vi "play_FXP_AFMss_LinearDistEst_singleAxis.vi"() -> ()   [LabVIEW 2017]
uses:
  fpga_VIs/fixed-point/typeDefs/FXPControlParams_distEst.ctl
  fpga_fp_interface_lib/fpga_interface_types/boolean_indicators.ctl
  <vilib>/Analysis/Matrix/Datatypes/RealMatrix.ctl
  <vilib>/userdefined/High Color/nirio_resource_hc.ctl
  <vilib>/Utility/error.llb/DialogType.ctl
  <vilib>/Analysis/Matrix/Numeric/Conversions/Matrix To Array - RM.vi
  <vilib>/Utility/file.llb/Read Delimited Spreadsheet (DBL).vi
  <vilib>/FPGAPlugInAG/cRIO-9082/niLvFpga_Open_cRIO-9082.vi
  <vilib>/rvi/interface/common/dynamic/niFpgaDynamicAddResources.vi
  <vilib>/FPGAPlugInAG/Dynamic/niLvFpga_Reset_Dynamic.vi
  <vilib>/rvi/interface/common/niFpgaWaitOnOcc.vi
  <vilib>/Utility/error.llb/Error Cluster From Error Code.vi
  <vilib>/rvi/errors/niLvFpgaAdjustHostInterfaceError.vi
  <vilib>/FPGAPlugInAG/Dynamic/niLvFpga_Run_Dynamic.vi
  <vilib>/RVI Host/nirviSupport.llb/nirviErrorClusterFromErrorCode.vi
  fpga_fp_interface_lib/write_FP_data_to_fpga.vi
  fpga_fp_interface_lib/acquire_FXP_18-5_FIFO_1.vi
  <vilib>/Utility/file.llb/Write To Spreadsheet File (DBL).vi
  <vilib>/Analysis/Matrix/Numeric/Conversions/Array To Matrix - RA2.vi
  <vilib>/FPGAPlugInAG/Dynamic/niLvFpga_Close_Dynamic.vi
  <vilib>/rvi/interface/nirviOpenFPGA/nirviOpenFPGA.xnode
  FPGA Bitfiles/XYpeizocontrol_FPGA_FXPAFMssLinearDistEst_singleAxis.lvbitx
  <vilib>/rvi/interface/nirviMethod/nirviMethod.xnode
  <vilib>/rvi/interface/nirviReadWriteControl/nirviReadWriteControl.xnode
  <vilib>/rvi/interface/nirviCloseFPGA/nirviCloseFPGA.xnode
  <vilib>/rvi/errors/niLvFpgaMergeErrorWithErrorCode.vi
  <vilib>/rvi/interface/Simulation/niFpgaSimulationCallBeginRW.vi
  <vilib>/rvi/interface/nirviMethod/StockFPGA_InlinedMethodWaitForSingleIRQ.vi
  <vilib>/FPGAPlugInAG/Dynamic/niLvFpga_WaitOnIrq_Dynamic.vi
  <vilib>/FPGAPlugInAG/Dynamic/niLvFpga_AcknowledgeIrq_Dynamic.vi
  <vilib>/FPGAPlugInAG/Dynamic/niLvFpga_ConfigureFifo_Dynamic.vi
  <vilib>/Analysis/Matrix/NI_Matrix.lvlib
  <vilib>/FPGAPlugInAG/Dynamic/niLvFpga_WriteFifo_Dynamic.vi
  labview/utils_lib/utils.lvlib
  NiFpgaLv.dll
panel:
  out "elements left":i32=1
  in  "N_hyst":i32
  in  "w_s":T1
  in  "r_s":T1
  in  "TF Order":i32
  in  "den":T1
  in  "num":T1
  in  "Tab Control":T2(tab)
  in  "traj_path":path=path "Z:/mpc-journal/step-exps/traj_data.csv"
  in  "TsTicks":i32=1600
  in  "umax":dbl=1.0 format="%#_13g"
  in  "ymax":dbl=4.0 format="%#_13g"
  in  "Iters":i32=25
  in  "SettleTicks":i32=10
  in  "dry_run":bool=TRUE
  in  "control_data_path":path=path "Z:/mpc-journal/step-exps/FXP_lin_Controls01.csv"
  in  "outputDataPath":path=path "Z:/mpc-journal/step-exps/expOut_multiAxis_tmp.csv"
  out "ControlParams":T3={"umax"=3.0, "Ns_obs/cntrl"=0, "ref_f_VEC"=[0.0, 0.0], "du_max"=0.0}
  in  "ABORT":bool
  out "XY Graph":cluster{dbl[], "2D Data Out":dbl[]}[](graph)
  in  "read_file":bool=TRUE
  in  "All_matrix":T1
  in  "Ns_obs/cntrl":u8=21
  in  "yref":T1
  in  "du_max":dbl=1.0 format="%#_13g"
  out "AllMatrix":dbl[](array[numeric])
  out "ControlMatrices":T4
  out "result_data":T1
  out "boolean  indicators":T5
  out "error out":errorcluster
  out "Empty Elements Remaining":u32
  out "size(s)":i32[](array[numeric])
  out "u_k out":fxp<+/-,32,5>
  # "NOTE: Ns is the number of states in the plant. The number of states in the \nobserver is Ns+1. Thus, for B, L, C, and A, we use NS+1. For K and Xss, we use Ns\nbecause the controller does not operate on the disturbance state, Xd."
  # "yk\nulin\ndu\nu_inv\nIpow\nX"
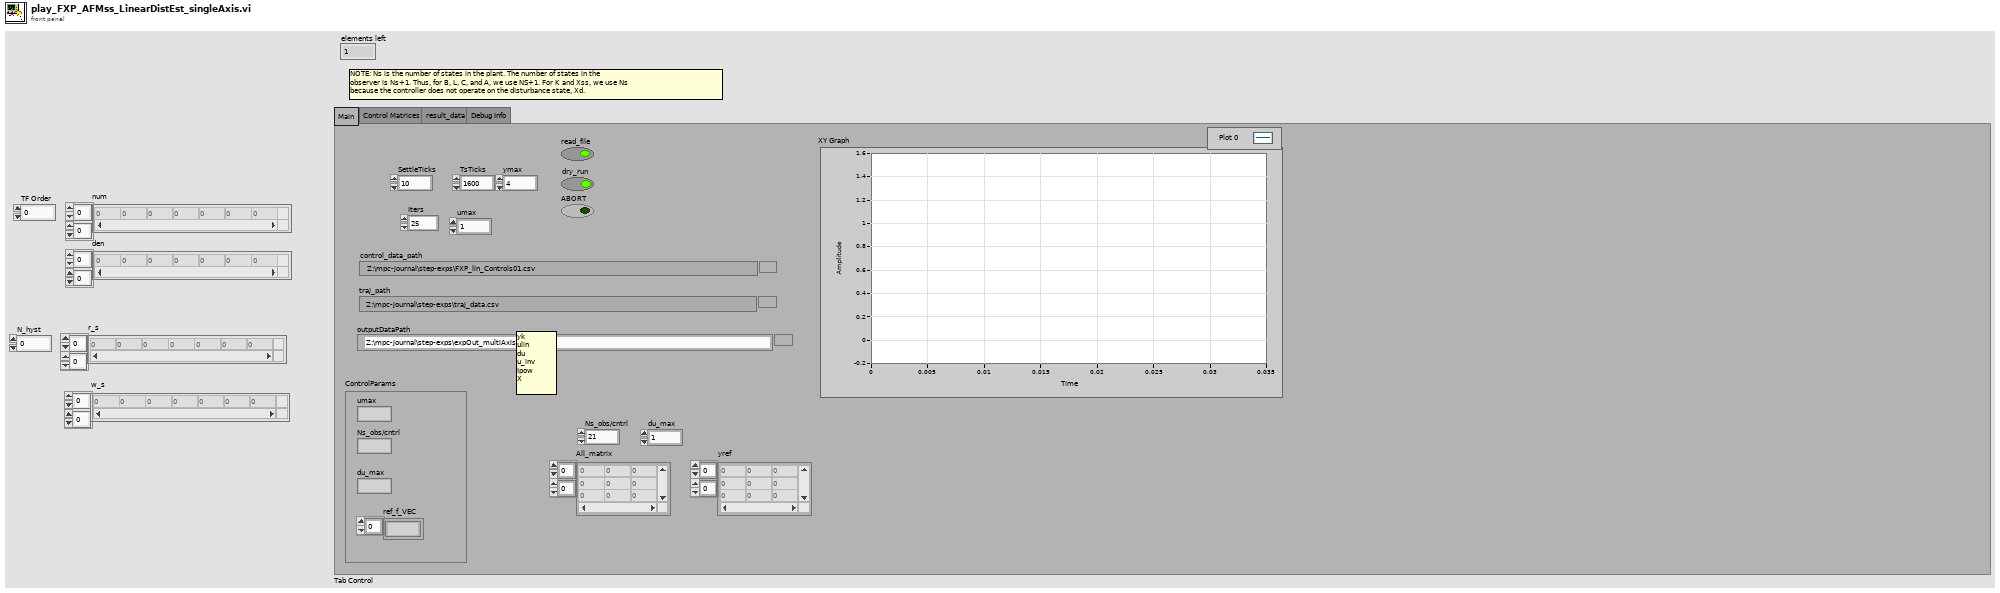
[diagram p1: front panel]
types:
  T1 = typedef "NI_Matrix.lvlib/RealMatrix.ctl" = dbl[][]
  T2 = enum32{"Main", "Control Matrices", "result_data", "Debug Info"}
  T3 = typedef "FXPControlParams_distEst.ctl" = cluster{"umax":fxp<+/-,18,5>, "Ns_obs/cntrl":u8, "ref_f_VEC":fxp<+/-,32,5>[], "du_max":fxp<+/-,18,5>}
  T4 = cluster{"Az":fxp<+/-,32,4>[][], "Bz":dbl[][], "Lz":dbl[][], "Kz":dbl[][], "NxNu":dbl[][]}
  T5 = typedef "boolean_indicators.ctl" = cluster{"unstable-z-traj":bool, "input fifo time-out":bool, "logging fifo timeout":bool, "scanning finished":bool, "unstable-x-traj":bool, "unstable-y-traj":bool, "ABORT":bool, "All Measurements Done":bool, "fpga_finished":bool}
  T6 = typedef "nirio_resource_hc.ctl" = tag
  T7 = typedef "ObserverMatrices.ctl" = cluster{"Az":fxp<+/-,32,4>[][], "Bz":dbl[][], "Lz":dbl[][], "Kz":dbl[][], "NxNu":dbl[][]}
  T8 = cluster{"unstable-z-traj":bool, "input fifo time-out":bool, "logging fifo timeout":bool, "scanning finished":bool, "unstable-x-traj":bool, "unstable-y-traj":bool, "ABORT":bool, "All Measurements Done":bool, "fpga_finished":bool}
  T9 = typedef "DialogType.ctl" = u16
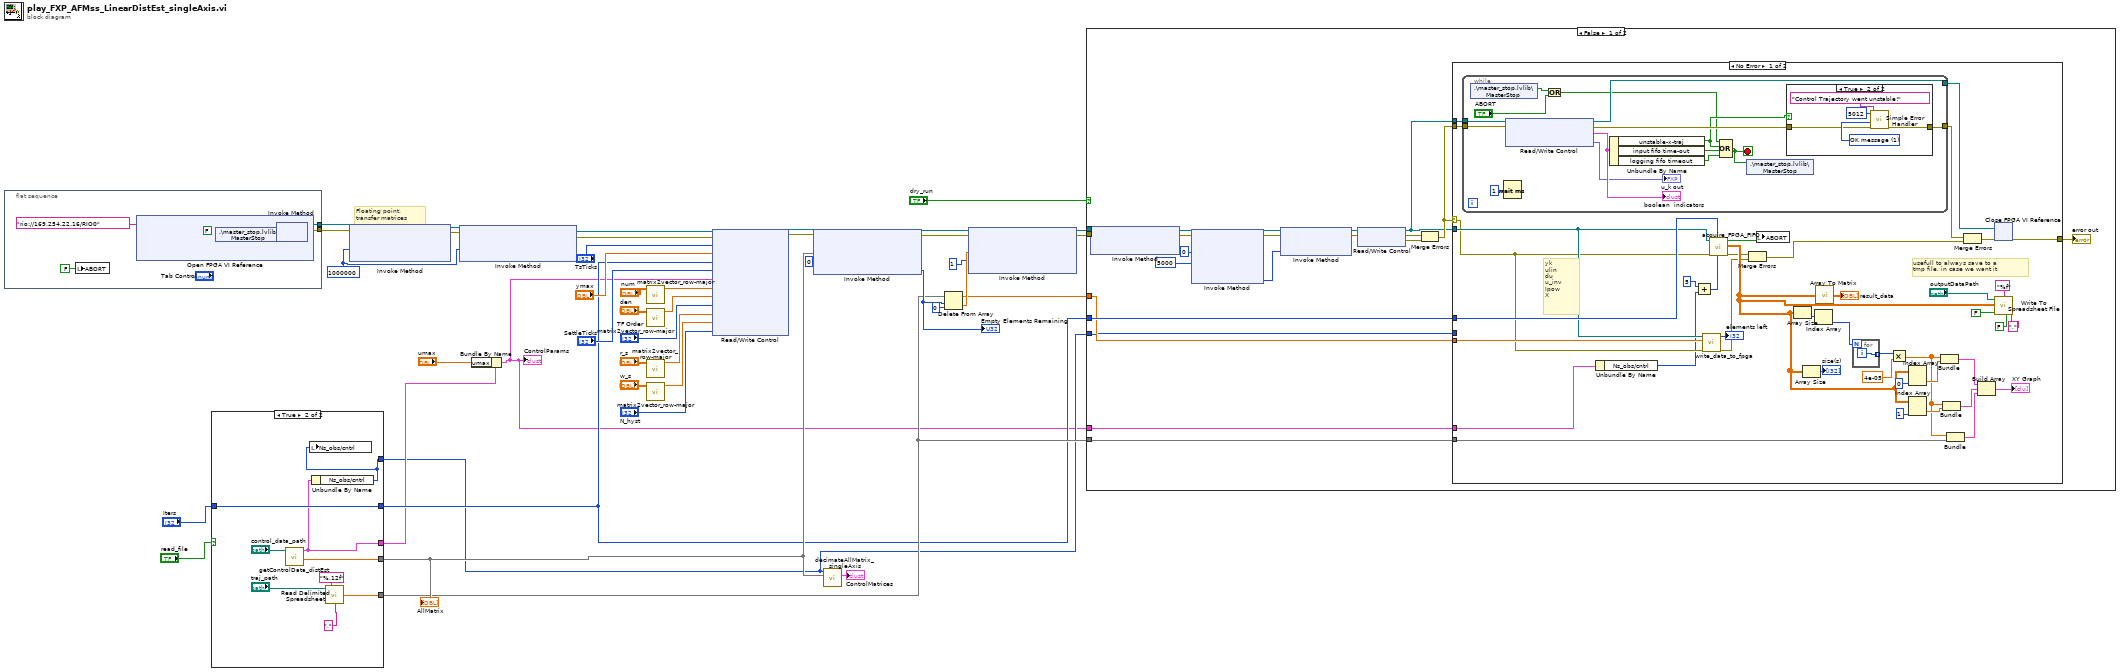
[diagram p0: block diagram]
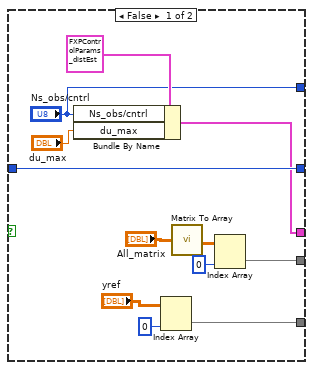
[diagram p2: hidden frame]
diagram:
  w2 = u32 1000000 ("Requested Depth")
  # "Floating point, \ntransfer matrices"
  n1 = flat-sequence {
    tunnel: [w50] -> w36
    tunnel: [w49] -> w35
    frame #0 {
      n2 = local write "ABORT"(FALSE) -> ()
      n3 = xnode "Open FPGA VI Reference"("resource name"=T6 "rio://169.254.22.16/RIO0") -> ("FPGA VI Reference Out"=w48:refnum<k20>, "error out"=w46:errorcluster)  [unwired: 1 in]
      n4 = shared-variable ".\\master_stop.lvlib\\MasterStop"(FALSE ("MasterStop"), error in=w46) -> (error out=w47:errorcluster)
      n5 = xnode "Invoke Method"("FPGA VI Reference In"=w48, "error in"=w47) -> ("FPGA VI Reference Out"=w50:refnum<k20>, "error out"=w49:errorcluster)
    }
  }
  n6 = case shown="True" "read_file" {
    tunnel: [w53 w65] -> w4
    tunnel: [w61 w71] -> w27
    tunnel: ["Ns_obs/cntrl" w64] -> w3
    tunnel: [w56 w68] -> w7
    tunnel: "Iters" -> [w59 w67]
    tunnel: [w59 w67] -> w5
    frame False {
      n7 = Bundle By Name(cluster=T3 {"umax"=3.0, "Ns_obs/cntrl"=0, "ref_f_VEC"=[0.0, 0.0], "du_max"=0.0} ("ControlParams 2"), "Ns_obs/cntrl"="Ns_obs/cntrl", "du_max"="du_max") -> (w53:T3)
      n8 = Index Array(array="yref", index (col)=0 ("disabled index (col)")) -> (element=w56:dbl[])  [unwired: 1 in]
      n9 = call-poly <vilib>:"Matrix To Array.vi"("Real Matrix"="All_matrix") -> ("Real 2D Array"=w62:dbl[][])
      n10 = Index Array(array=w62, index (col)=0 ("disabled index (col)")) -> (element=w61:dbl[])  [unwired: 1 in]
    }
    frame True {
      n11 = call "getControlData_distEst.vi"("system matricec path"="control_data_path") -> ("AllMatrix"=w71:dbl[], "ControlParams"=w65:T3)  [unwired: 6 in, 3 out]
      n12 = Unbundle By Name(w65) -> ("Ns_obs/cntrl"=w64:u8)
      n13 = local write "Ns_obs/cntrl"(w64) -> ()
      n14 = call-poly <vilib>:"Read Delimited Spreadsheet.vi"("file path (dialog if empty)"="traj_path", "format (%.3f)"="%.12f", "delimiter (\\t)"="," ("format (%.3f)")) -> ("first row"=w68:dbl[])  [unwired: 7 in, 5 out]
    }
  }
  "AllMatrix" <- w27
  n15 = xnode "Invoke Method"("FPGA VI Reference In"=w36, "error in"=w35, "Requested Depth"=w2) -> ("FPGA VI Reference Out"=w34:refnum<k20>, "error out"=w33:errorcluster)  [unwired: 1 out]
  n16 = xnode "Invoke Method"("FPGA VI Reference In"=w34, "error in"=w33, "Requested Depth"=w2) -> ("FPGA VI Reference Out"=w31:refnum<k20>, "error out"=w32:errorcluster)  [unwired: 1 out]
  n17 = Bundle By Name(cluster=w4, "umax"="umax") -> (w1:T3)
  "ControlParams" <- w1
  n18 = call "matrix2vector_row-major.vi"("Matrix"="num") -> ("vector"=w22:dbl[])  [unwired: 10 in]
  n19 = call "matrix2vector_row-major.vi"("Matrix"="den") -> ("vector"=w21:dbl[])  [unwired: 10 in]
  n20 = call "matrix2vector_row-major.vi"("Matrix"="r_s") -> ("vector"=w19:dbl[])  [unwired: 10 in]
  n21 = call "matrix2vector_row-major.vi"("Matrix"="w_s") -> ("vector"=w18:dbl[])  [unwired: 10 in]
  n22 = xnode "Read/Write Control"("FPGA VI Reference In"=w31, "error in"=w32, "TsTicks"="TsTicks", "ymax"="ymax", "iters"=w5, "Settle Ticks"="SettleTicks", "ControlParamsMpc"=w1, "Num"=w22, "Den"=w21, "TF Order"="TF Order", "r_s"=w19, "w_s"=w18, "N_hyst"="N_hyst") -> ("FPGA VI Reference Out"=w40:refnum<k20>, "error out"=w39:errorcluster)
  n23 = xnode "Invoke Method"("FPGA VI Reference In"=w40, "error in"=w39, "Data"=w27, "Timeout (ms)"=0) -> ("FPGA VI Reference Out"=w12:refnum<k20>, "error out"=w11:errorcluster, "Empty Elements Remaining"=w10:u32)
  "Empty Elements Remaining" <- w10
  n24 = call "decimateAllMatrix_singleAxis.vi"("AllMatrix"=w27, "NS_obs/cntrl"=w3) -> ("ControlMatrices"=→"ControlMatrices":T7)  [unwired: 8 in, 1 out]
  n25 = Delete From Array(array=w7, length=w10, index=0) -> (deleted portion=w16:dbl[], array with subset deleted=w8:dbl[])
  n26 = xnode "Invoke Method"("FPGA VI Reference In"=w12, "error in"=w11, "Data"=w16, "Timeout (ms)"=1) -> ("FPGA VI Reference Out"=w14:refnum<k20>, "error out"=w13:errorcluster)  [unwired: 1 out]
  n27 = case shown="False" "dry_run" {
    tunnel: w14 -> [w93 _]
    tunnel: w13 -> [w92 _]
    tunnel: w5 -> [w79 _]
    tunnel: w8 -> [w76 _]
    tunnel: w7 -> [w75 _]
    tunnel: w3 -> [w74 _]
    tunnel: w1 -> [w73 _]
    frame False {
      n28 = xnode "Invoke Method"("FPGA VI Reference In"=w93, "error in"=w92) -> ("FPGA VI Reference Out"=w83:refnum<k20>, "error out"=w84:errorcluster)  [unwired: 1 in]
      n29 = xnode "Invoke Method"("FPGA VI Reference In"=w83, "error in"=w84, "IRQ Number(s)"=0, "Timeout (ms)"=5000) -> ("FPGA VI Reference Out"=w89:refnum<k20>, "error out"=w90:errorcluster, "IRQ(s) Asserted"=w86:i32)  [unwired: 1 out]
      n30 = xnode "Invoke Method"("FPGA VI Reference In"=w89, "error in"=w90, "IRQ Number(s)"=w86) -> ("FPGA VI Reference Out"=w88:refnum<k20>, "error out"=w87:errorcluster)
      n31 = xnode "Read/Write Control"("FPGA VI Reference In"=w88, "error in"=w87) -> ("FPGA VI Reference Out"=w77:refnum<k20>, "error out"=w91:errorcluster, "Error Out"=w81:errorcluster)
      n32 = Merge Errors(w91, w81) -> (w78:errorcluster)
      n33 = case shown="No Error" w78 {
        selector: w78 -> [w107 w157]
        tunnel: [w133 w157] -> w80
        tunnel: w77 -> [w132 _]
        tunnel: w78 -> [w131 _]
        tunnel: w79 -> [w128 _]
        tunnel: w77 -> [w109 _]
        tunnel: w76 -> [w108 _]
        tunnel: w75 -> [w100 _]
        tunnel: w74 -> [_ _]
        tunnel: w73 -> [w97 _]
        frame No Error {
          # "yk\nulin\ndu\nu_inv\nIpow\nX"
          # "usefull to always save to a \ntmp file, in case we want it"
          n34 = while {
            tunnel: w132 -> [w149]
            tunnel: w131 -> [w148]
            tunnel: [w146] -> w130
            tunnel: [w145] -> w129
            stop <- w144 stop-if-true
            n35 = shared-variable ".\\master_stop.lvlib\\MasterStop"() -> (w139:bool)  [unwired: 1 in, 1 out]
            n36 = Wait (ms)(milliseconds to wait=u32 1) -> ()  [unwired: 1 out]
            n37 = xnode "Read/Write Control"("FPGA VI Reference In"=w149, "error in"=w148) -> ("FPGA VI Reference Out"=w145:refnum<k20>, "error out"=w147:errorcluster, "boolean  indicators"=w143:T8, "u_k"=→"u_k out":fxp<+/-,32,5>)
            "boolean  indicators" <- w143
            n38 = Or(x=w139, y="ABORT") -> (x .or. y?=w137:bool)
            n39 = Unbundle By Name(w143) -> ("unstable-x-traj"=w141:bool, "input fifo time-out"=w142:bool, "logging fifo timeout"=w140:bool)
            n40 = Compound Arithmetic op=OR(w137, w141, w142, w140) -> (w144:bool)
            n41 = shared-variable ".\\master_stop.lvlib\\MasterStop"(w144) -> ()  [unwired: 1 in, 1 out]
            n42 = case shown="True" w141 {
              tunnel: w147 -> [w151 w153]
              tunnel: [w151 w152] -> w146
              frame False {
              }
              frame True {
                w156 = T9 1 items=["no dialog", "OK message", "continue or stop message", "OK message + warnings", "continue/stop + warnings"] ("type of dialog (OK msg:1)")
                n43 = call <vilib>:"Simple Error Handler.vi"("error code (no error:0)"=5012, "error source (\" \")"="Control Trajectory went unstable!" ("error source (\" \")"), "type of dialog (OK msg:1)"=w156, "error in (no error)"=w153) -> ("error out"=w152:errorcluster)  [unwired: 1 in, 4 out]
              }
            }
          }
          n44 = Unbundle By Name(w97) -> ("Ns_obs/cntrl"=w94:u8)
          n45 = Add(x=u8 5 ("y"), y=w94) -> (x+y=w96:u8)
          n46 = call-poly "write_data_to_fpga.vi"("error in"=w107, "all rows"=w108, "FPGA Interface"=w109) -> ("error out"=w104:errorcluster, "elements left"=→"elements left":i32)  [unwired: 7 in]
          n47 = call-poly "acquire_FPGA_FIFO.vi"("numChannels"=w96, "Iters"=w128, "error in"=w107, "FPGA Interface"=w109) -> ("error out"=w106:errorcluster, "2D Data Out"=w125:dbl[][], "acquisition done"=w127:bool)  [unwired: 3 in, 2 out]
          n48 = Merge Errors(w106, w104) -> (w105:errorcluster)
          n49 = local write "ABORT"(w127) -> ()
          n50 = Array Size(array=w125) -> (size(s)=w121:i32[])
          n51 = Array Size(array=w125) -> (size(s)=→"size(s)":i32[])
          n52 = Index Array(array=w121) -> (element=w120:i32)  [unwired: 1 in]
          n53 = call-poly <vilib>:"Array To Matrix.vi"("Real 2D Array"=w125) -> ("Real Matrix"=→"result_data":T1)
          n54 = for {
            N: w120 -> [_]
            tunnel: [w135] -> w119 mode=indexing
            i -> [w135]
          }
          n55 = Multiply(x=w119, y=4e-05) -> (x*y=w102:dbl[])
          n56 = Index Array(array=w125, index (col)=0 ("disabled index (col)")) -> (element=w117:dbl[])  [unwired: 1 in]
          n57 = Index Array(array=w125, index (col)=1 ("index (row)")) -> (element=w116:dbl[])  [unwired: 1 in]
          n58 = Bundle(w102, "2D Data Out"=w117) -> (w114:cluster{dbl[], "2D Data Out":dbl[]})  [unwired: 1 in]
          n59 = Bundle(w102, "2D Data Out"=w116) -> (w115:cluster{dbl[], "2D Data Out":dbl[]})  [unwired: 1 in]
          n60 = Bundle(w102, "first row"=w100) -> (w101:cluster{dbl[], "first row":dbl[]})  [unwired: 1 in]
          n61 = Merge Errors(w130, w105) -> (w134:errorcluster)
          n62 = Build Array(w114, w115, w101) -> (→"XY Graph":cluster{dbl[], "first row":dbl[]}[])
          n63 = xnode "Close FPGA VI Reference"("FPGA VI Reference In"=w129, "error in"=w134) -> ("error out"=w133:errorcluster)
          n64 = call-poly <vilib>:"Write To Spreadsheet File.vi"("delimiter (\\t)"=",", "transpose? (no:F)"=FALSE, "format (%.3f)"="%f", "append to file? (new file:F)"=FALSE, "2D data"=w125, "file path (dialog if empty)"="outputDataPath") -> ()  [unwired: 2 in, 1 out]
        }
        frame Error {
        }
      }
      "error out" <- w80
    }
    frame True {
    }
  }
